vi "PAQaveraging.vi"(5 "Size":i32, 6 "Crossover?":bool, 7 "Index":i32, 8 "error in (no error)":errorcluster, 9 "TAGs":i32[](array[numeric]), 10 "TAGdata":T2(array[cluster]), 11 "Length":i32) -> (0 "error out":errorcluster, 2 "Results":T1 {"status" format="%x"; "min" format="%.2f"; "max" format="%.2f"; "data" format="%.2f"})   [LabVIEW 2020, in "Sgraph_lib_V1.lvlib" / "FAMM.lvclass"]
doc: "Perform Averaging and min/max calculations over a given data set"
uses:
  FAMM.lvclass
  <vilib>/Analysis/baseanly.llb/Mean (DBL).vi
  <vilib>/Analysis/NI_AALBase.lvlib
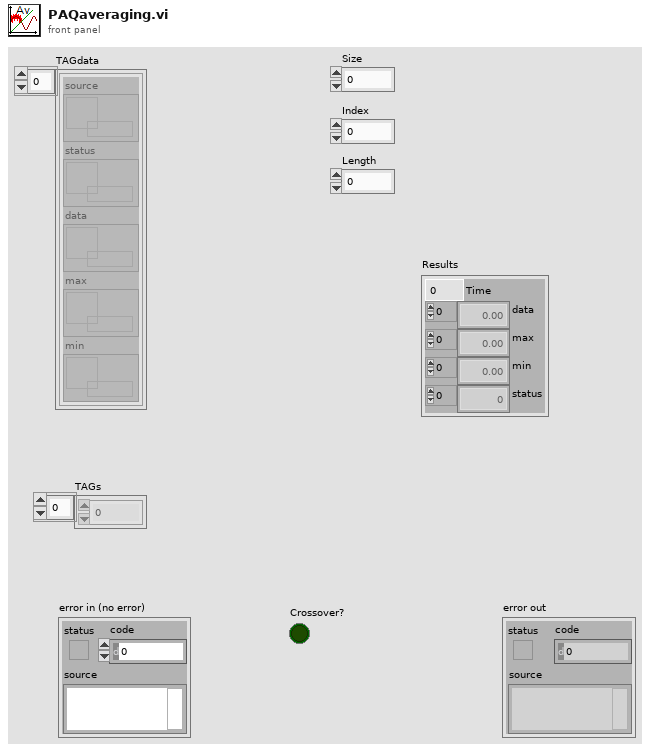
[diagram p1: front panel]
types:
  T1 = cluster{"Time":dbl, "data":dbl[], "max":dbl[], "min":dbl[], "status":u32[]}
  T2 = cluster{"source":refnum<data-value>, "status":refnum<data-value>, "data":refnum<data-value>, "max":refnum<data-value>, "min":refnum<data-value>}[]
  T3 = cluster{"source":refnum<data-value>, "status":refnum<data-value>, "data":refnum<data-value>, "max":refnum<data-value>, "min":refnum<data-value>}
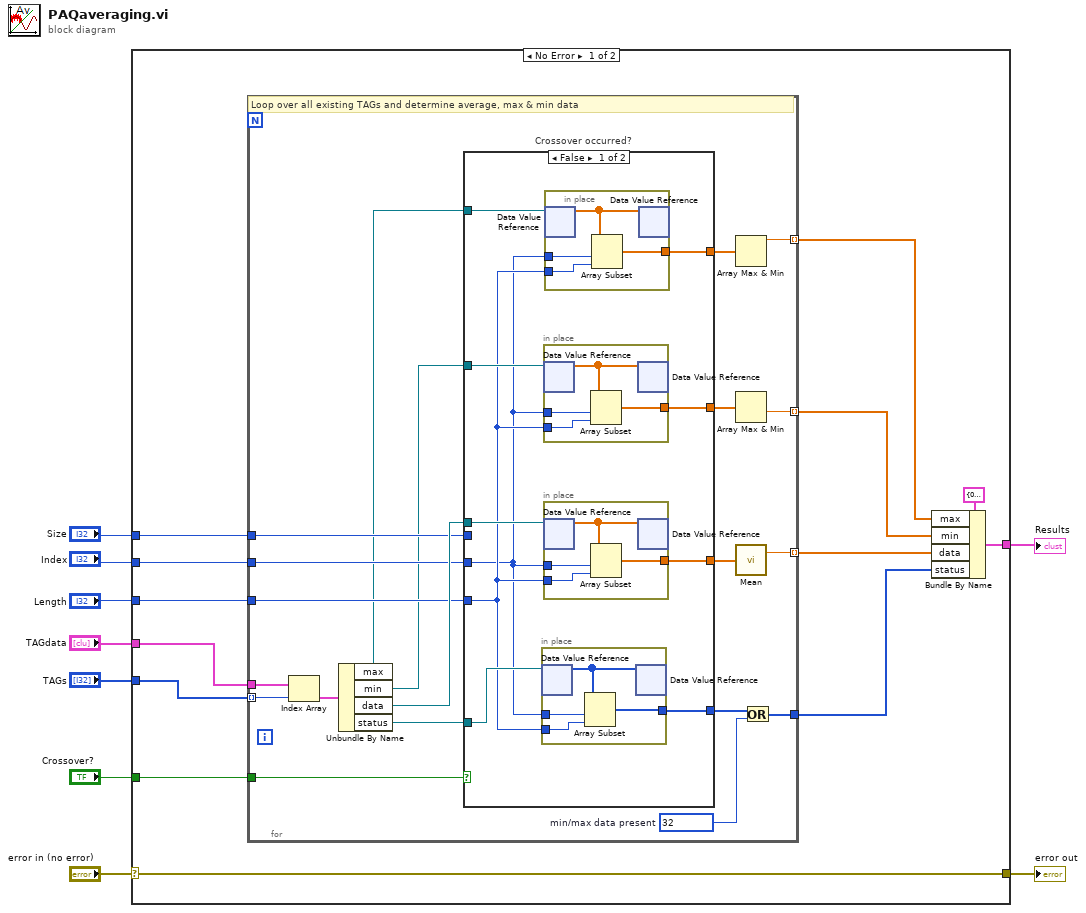
[diagram p0: block diagram]
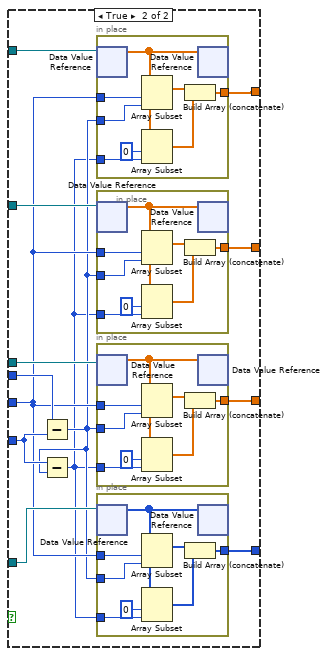
[diagram p2: hidden frame]
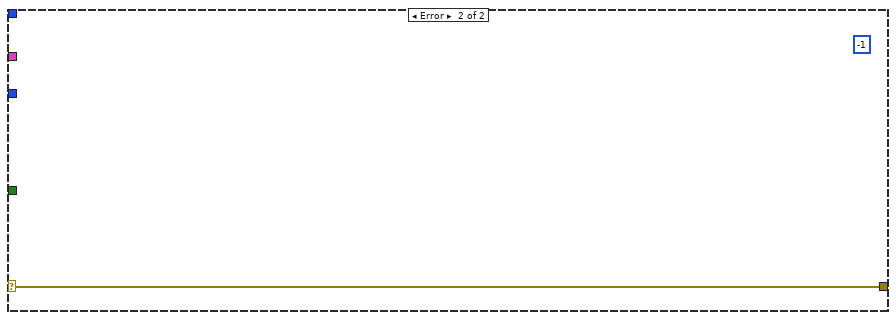
[diagram p3: hidden frame]
diagram:
  n1 = case shown="No Error" "error in (no error)" {
    selector: "error in (no error)" -> [w13 w114]
    tunnel: [w13 w114] -> w8
    tunnel: "Crossover?" -> [w22 _]
    tunnel: "Size" -> [w21 _]
    tunnel: "Index" -> [w20 _]
    tunnel: "Length" -> [w19 _]
    tunnel: "TAGs" -> [w18 _]
    tunnel: "TAGdata" -> [w17 _]
    tunnel: [w14 _] -> w1
    frame No Error {
      n2 = for {
        tunnel: w18 -> [w40] mode=indexing
        tunnel: w17 -> [w41]
        tunnel: w20 -> [w37]
        tunnel: w19 -> [w36]
        tunnel: [w34] -> w10 mode=indexing
        tunnel: [w26] -> w12 mode=indexing
        tunnel: [w33] -> w15
        tunnel: w22 -> [w32]
        tunnel: w21 -> [w31]
        tunnel: [w25] -> w11 mode=indexing
        w24 = u32 32  # min/max data present
        # "Loop over all existing TAGs and determine average, max & min data"
        n3 = Index Array(array=w41, index=w40) -> (element=w39:T3)
        n4 = Unbundle By Name(w39) -> ("max"=w30:refnum<data-value>, "min"=w29:refnum<data-value>, "data"=w42:refnum<data-value>, "status"=w38:refnum<data-value>)
        n5 = case "Crossover occurred?" shown="False" w32 {
          tunnel: w42 -> [w52 w81]
          tunnel: w38 -> [w51 w80]
          tunnel: w37 -> [w43 w71]
          tunnel: w36 -> [w46 w78]
          tunnel: [w50 w77] -> w23
          tunnel: [w49 w76] -> w35
          tunnel: w31 -> [_ w79]
          tunnel: w30 -> [w48 w75]
          tunnel: w29 -> [w47 w74]
          tunnel: [w45 w73] -> w28
          tunnel: [w44 w72] -> w27
          frame False {
            n6 = in-place {
              in-place-border: w43 -> [w63]
              in-place-border: w46 -> [w62]
              in-place-border: [w61] -> w49
              n7 = in-place-dvr #1(w51) -> (w64:u32[])  [unwired: 1 out]
              n8 = Array Subset(array=w64, index=w63, length=w62) -> (w61:u32[])
              n9 = in-place-dvr #1(w64) -> ()  [unwired: 2 out]
            }
            n10 = in-place {
              in-place-border: w43 -> [w59]
              in-place-border: w46 -> [w58]
              in-place-border: [w57] -> w44
              n11 = in-place-dvr #2(w47) -> (w60:dbl[])  [unwired: 1 out]
              n12 = Array Subset(array=w60, index=w59, length=w58) -> (w57:dbl[])
              n13 = in-place-dvr #2(w60) -> ()  [unwired: 2 out]
            }
            n14 = in-place {
              in-place-border: w43 -> [w67]
              in-place-border: w46 -> [w66]
              in-place-border: [w65] -> w50
              n15 = in-place-dvr #3(w52) -> (w68:dbl[])  [unwired: 1 out]
              n16 = Array Subset(array=w68, index=w67, length=w66) -> (w65:dbl[])
              n17 = in-place-dvr #3(w68) -> ()  [unwired: 2 out]
            }
            n18 = in-place {
              in-place-border: w43 -> [w55]
              in-place-border: w46 -> [w54]
              in-place-border: [w53] -> w45
              n19 = in-place-dvr #4(w48) -> (w56:dbl[])  [unwired: 1 out]
              n20 = Array Subset(array=w56, index=w55, length=w54) -> (w53:dbl[])
              n21 = in-place-dvr #4(w56) -> ()  [unwired: 2 out]
            }
          }
          frame True {
            n22 = Subtract(x=w79, y=w78) -> (x-y=w70:i32)
            n23 = Subtract(x=w78, y=w70) -> (x-y=w69:i32)
            n24 = in-place {
              in-place-border: w71 -> [w89]
              in-place-border: w70 -> [w88]
              in-place-border: w69 -> [w85]
              in-place-border: [w82] -> w73
              n25 = in-place-dvr #5(w75) -> (w87:dbl[])  [unwired: 1 out]
              n26 = Array Subset(array=w87, index=w89, length=w88) -> (w84:dbl[])
              n27 = Array Subset(array=w87, index=0, length=w85) -> (w83:dbl[])
              n28 = Build Array (concatenate)(w84, w83) -> (w82:dbl[])
              n29 = in-place-dvr #5(w87) -> ()  [unwired: 2 out]
            }
            n30 = in-place {
              in-place-border: w71 -> [w97]
              in-place-border: w70 -> [w96]
              in-place-border: w69 -> [w93]
              in-place-border: [w90] -> w72
              n31 = in-place-dvr #6(w74) -> (w95:dbl[])  [unwired: 1 out]
              n32 = Array Subset(array=w95, index=w97, length=w96) -> (w92:dbl[])
              n33 = Array Subset(array=w95, index=0, length=w93) -> (w91:dbl[])
              n34 = Build Array (concatenate)(w92, w91) -> (w90:dbl[])
              n35 = in-place-dvr #6(w95) -> ()  [unwired: 2 out]
            }
            n36 = in-place {
              in-place-border: w71 -> [w113]
              in-place-border: w70 -> [w112]
              in-place-border: w69 -> [w109]
              in-place-border: [w106] -> w77
              n37 = in-place-dvr #7(w81) -> (w111:dbl[])  [unwired: 1 out]
              n38 = Array Subset(array=w111, index=w113, length=w112) -> (w108:dbl[])
              n39 = Array Subset(array=w111, index=0, length=w109) -> (w107:dbl[])
              n40 = Build Array (concatenate)(w108, w107) -> (w106:dbl[])
              n41 = in-place-dvr #7(w111) -> ()  [unwired: 2 out]
            }
            n42 = in-place {
              in-place-border: w71 -> [w105]
              in-place-border: w70 -> [w104]
              in-place-border: w69 -> [w101]
              in-place-border: [w98] -> w76
              n43 = in-place-dvr #8(w80) -> (w103:u32[])  [unwired: 1 out]
              n44 = Array Subset(array=w103, index=w105, length=w104) -> (w100:u32[])
              n45 = Array Subset(array=w103, index=0, length=w101) -> (w99:u32[])
              n46 = Build Array (concatenate)(w100, w99) -> (w98:u32[])
              n47 = in-place-dvr #8(w103) -> ()  [unwired: 2 out]
            }
          }
        }
        n48 = Array Max & Min(array=w28) -> (max value=w26:dbl)  [unwired: 3 out]
        n49 = Array Max & Min(array=w27) -> (min value=w25:dbl)  [unwired: 3 out]
        n50 = call-poly <vilib>:"Mean.vi"("X"=w23) -> ("mean"=w34:dbl)  [unwired: 1 out]
        n51 = Or(x=w35, y=w24) -> (x .or. y?=w33:u32[])
      }
      n52 = Bundle By Name(cluster=T1 {"Time"=0.0, "data"=[], "max"=[], "min"=[], "status"=[]} ("Results"), "max"=w12, "min"=w11, "data"=w10, "status"=w15) -> (w14:T1)
    }
    frame Error {
      (unwired) -1 ("Index")
    }
  }
  "Results" <- w1
  "error out" <- w8
